vi "AMC Send Message.vi"(4 "Acknowledge Message (F)":bool, 5 "Receiver Host":string, 6 "Source Process":string, 7 "Receiver Process":string, 8 "error in (no error)":errorcluster, 9 "Priority Message (F)":bool, 10 "Message":T1, 11 "Message Queue in":T3) -> (0 "error out":errorcluster, 3 "Message Queue out":T3)   [LabVIEW 2009]
doc: "This VI is used for compatibility with previous versions of the AMC library. Use the AMC VIs located in the <b>Data Communication >> Asynchronous Message Communication</b> palette."
uses:
  Message Queue.ctl
  Message.ctl
  <vilib>/NI/Tools/Keyed Array/KeyedArray.ctl
  AMC.lvlib
  <vilib>/NI/Tools/Keyed Array/Tools_KeyedArray.lvlib
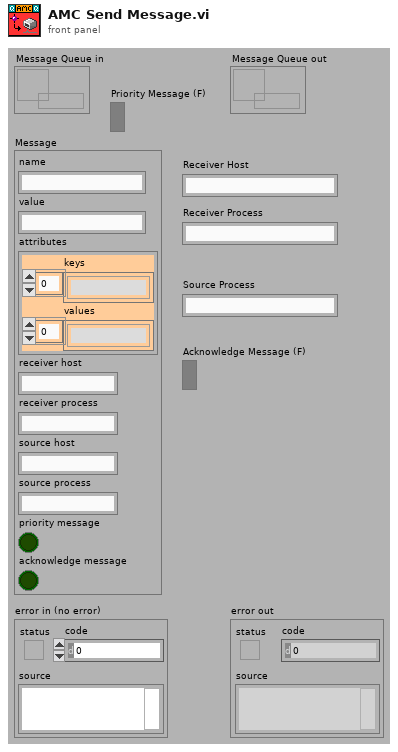
[diagram p1: front panel]
types:
  T1 = typedef "AMC.lvlib/Message.ctl" = cluster{"name":string, "value":string, "attributes":T2, "receiver host":string, "receiver process":string, "source host":string, "source process":string, "priority message":bool, "acknowledge message":bool}
  T2 = typedef "Tools_KeyedArray.lvlib/KeyedArray.ctl" = cluster{"keys":string[], "values":string[]}
  T3 = typedef "AMC.lvlib/Message Queue.ctl" = refnum<queue>
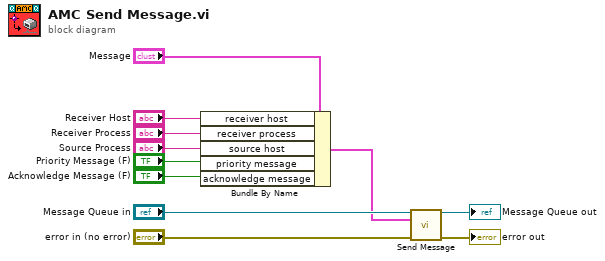
[diagram p0: block diagram]
diagram:
  n1 = Bundle By Name(cluster="Message", "receiver host"="Receiver Host", "receiver process"="Receiver Process", "source host"="Source Process", "priority message"="Priority Message (F)", "acknowledge message"="Acknowledge Message (F)") -> (w1:T1)
  n2 = call "Send Message.vi"("message queue in"="Message Queue in", "message"=w1, "error in"="error in (no error)") -> ("message queue out"=→"Message Queue out":T3, "error out"=→"error out":errorcluster)  [unwired: 10 in, 1 out]
